vi "measure.vi"(11 "Qube":refnum<class "System.lvclass">) -> (3 "Qube":refnum<class "System.lvclass">)   [LabVIEW 2021, in "System.lvclass"]
uses:
  System.lvclass
  System.lvclass/System.ctl
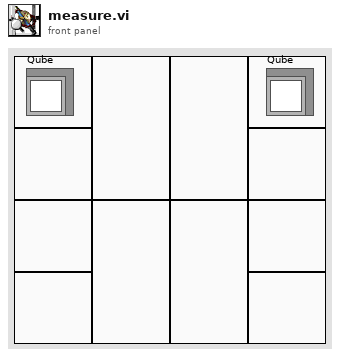
[diagram p1: front panel]
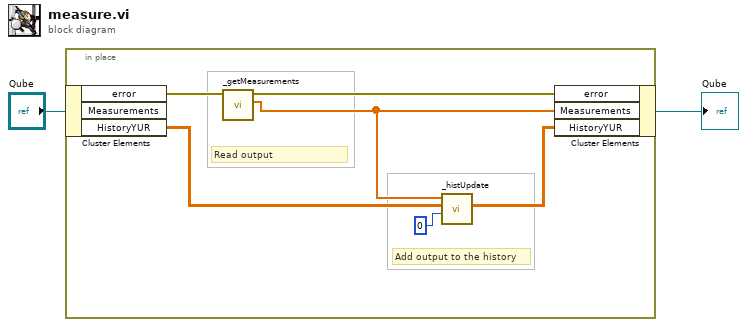
[diagram p0: block diagram]
diagram:
  n1 = in-place {
    # "Read output"
    # "Add output to the history"
    n2 = in-place-cluster #1("Qube") -> ("error"=w8:errorcluster, "HistoryYUR"=w5:dbl[][][])  [unwired: 1 out]
    n3 = call "_getMeasurements.vi"("error in (no error)"=w8) -> ("pry"=w4:dbl[], "error out"=w7:errorcluster)  [unwired: 9 in]
    n4 = call "_histUpdate.vi"("Y:0-U:1-R:2"=0, "History In"=w5, "pry"=w4) -> ("History Out"=w3:dbl[][][])  [unwired: 8 in]
    n5 = in-place-cluster #1("error"=w7, "Measurements"=w4, "HistoryYUR"=w3) -> (→"Qube":refnum<class "System.lvclass">)
  }
